vi "Get Head Impulse Sheet.vi"(8 "error in (no error)":errorcluster, 11 "Excel Logger in":refnum<class "Excel Logger.lvclass">) -> (0 "error out":errorcluster, 2 "Head Impulse":refnum<class "Data Analyser Report.lvclass">, 3 "Excel Logger out":refnum<class "Excel Logger.lvclass">)   [LabVIEW 2016, in "Excel Logger.lvclass"]
uses:
  Excel Logger.lvclass
  Data Analyser Report/Data Analyser Report.lvclass
  Excel Logger.lvclass/Excel Logger.ctl
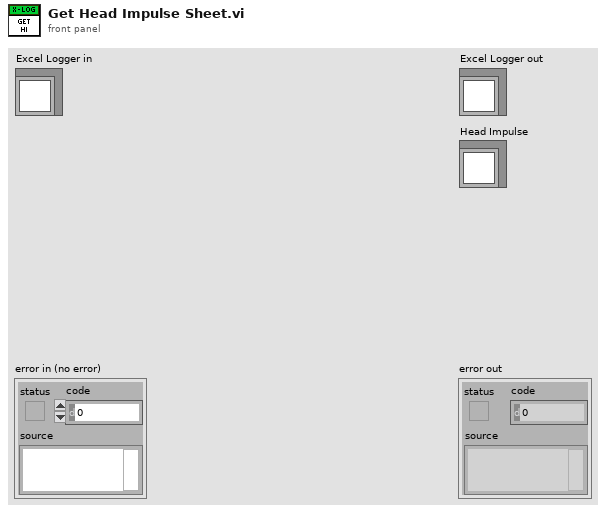
[diagram p1: front panel]
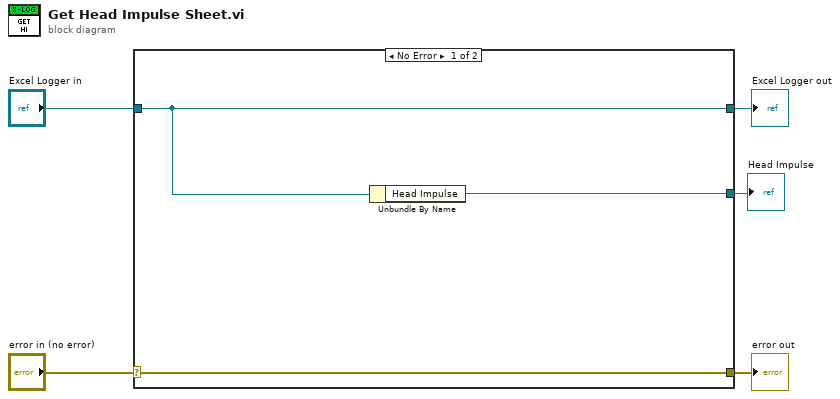
[diagram p0: block diagram]
diagram:
  n1 = case shown="No Error" "error in (no error)" {
    selector: "error in (no error)" -> [w8 w10]
    tunnel: [w8 w10] -> w4
    tunnel: [w7 w9] -> w2
    tunnel: "Excel Logger in" -> [w7 w9]
    tunnel: [w6 _] -> w1
    frame No Error {
      n2 = Unbundle By Name(w7) -> ("Head Impulse"=w6:refnum<class "Data Analyser Report.lvclass">)
    }
    frame Error {
    }
  }
  "error out" <- w4
  "Excel Logger out" <- w2
  "Head Impulse" <- w1
